vi "SendMessage_Poly.vi"   [LabVIEW 2013, in "CLM_PriorityLocalMessage.lvclass"]
uses:
  CLM_PriorityLocalMessage.lvclass
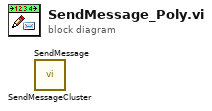
[diagram p0: block diagram]
diagram:
  n1 = call "SendMessageCluster.vi"() -> ()  [unwired: 8 in, 4 out]
  n2 = call "SendMessage.vi"() -> ()  [unwired: 8 in, 4 out]
